vi "CreatePublicEvents.vi"(8 "error in (no error)":errorcluster, 11 "Camera":refnum<class "Camera.lvclass">) -> (0 "error out":errorcluster, 3 "Camera out":refnum<class "Camera.lvclass">)   [LabVIEW 2015, in "Camera.lvclass"]
doc: "---------------------------------------------------------------\nJKI State Machine Objects™\nhttp://jki.net/state-machine-objects/\nCopyright (C) 2005-2015, JKI <info@jki.net>\nALL RIGHTS RESERVEDJKI State Machine Objects (SMO) 1.0.0.5\nJKI - JKI\nCopyright (c) 2016, JKI"
uses:
  Camera.lvclass
  Camera.lvclass/Camera.ctl
  Typedefs/PublicEvents--Camera.NewImage.ctl
  <vilib>/JKI/JKI SMO/SMO/SMO.lvclass
panel:
  # "For instructions on how to use the JKI State Machine Objects, examples and video tutorials, visit:\nhttp://jki.net/state-machine-objects/\n\nJKI State Machine Objects™\nhttp://jki.net/state-machine-objects/\nCopyright (C) 2005-2015, JKI <info@jki.net>\nALL RIGHTS RESERVED"
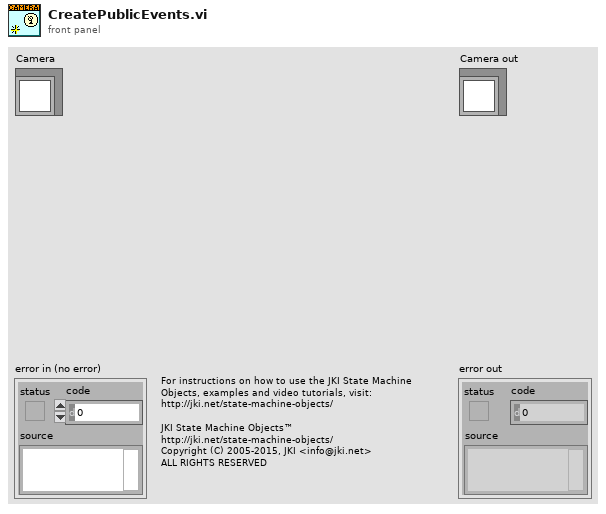
[diagram p1: front panel]
types:
  T1 = typedef "Camera.lvclass/PrivateData--Ref.ctl" = refnum<data-value>
  T2 = typedef "Camera.lvclass/PublicEvents--Camera.NewImage.ctl" = i32
  T3 = typedef "Camera.lvclass/PrivateData--Cluster.ctl" = cluster{"Public Events":T4, "Protected Events":T5, "Private Events":T6, "Dependencies":T7}
  T4 = typedef "Camera.lvclass/PublicEvents--Cluster.ctl" = cluster{"Value Changed":refnum<user-event>, "NewImage":refnum<user-event>, "ImageSaved":refnum<user-event>}
  T5 = typedef "Camera.lvclass/ProtectedEvents--Cluster.ctl" = cluster{"placeholder":refnum<user-event>}
  T6 = typedef "Camera.lvclass/PrivateEvents--Cluster.ctl" = cluster{"New Value":refnum<user-event>, "Grab Image":refnum<user-event>, "Save Image":refnum<user-event>, "Get Image":refnum<user-event>}
  T7 = typedef "Camera.Simulated.lvclass/Dependencies--Cluster.ctl" = cluster{"CircularBuffer.ImageData":refnum<class "CircularBuffer.ImageData.lvclass">}
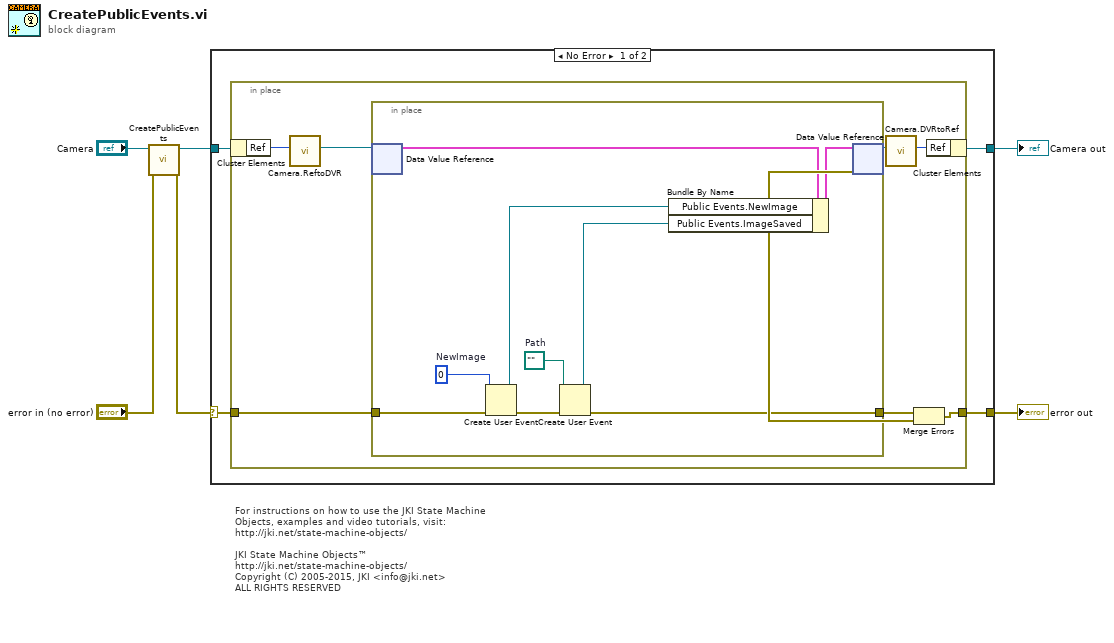
[diagram p0: block diagram]
diagram:
  # "For instructions on how to use the JKI State Machine Objects, examples and video tutorials, visit:\nhttp://jki.net/state-machine-objects/\n\nJKI State Machine Objects™\nhttp://jki.net/state-machine-objects/\nCopyright (C) 2005-2015, JKI <info@jki.net>\nALL RIGHTS RESERVED"
  n1 = call-parent "CreatePublicEvents.vi"("error in (no error)"="error in (no error)", "SMO"="Camera") -> ("error out"=w1:errorcluster, "SMO out"=w3:refnum<class "Camera.lvclass">)  [unwired: 8 in]
  n2 = case shown="No Error" w1 {
    selector: w1 -> [w8 w29]
    tunnel: [w7 w29] -> w5
    tunnel: [w9 w28] -> w6
    tunnel: w3 -> [w10 w28]
    frame No Error {
      n3 = in-place {
        in-place-border: w8 -> [w18]
        in-place-border: [w15] -> w7
        n4 = in-place-cluster #1(w10) -> ("Ref"=w14:u32)
        n5 = call "Camera.ReftoDVR.vi"("Ref"=w14) -> ("Ref"=w13:T1)  [unwired: 10 in]
        n6 = in-place {
          in-place-border: w18 -> [w19]
          in-place-border: [w22] -> w17
          w20 = path ""  # Path
          w24 = T2 0  # NewImage
          n7 = in-place-dvr #2(w13) -> (w26:T3)  [unwired: 1 out]
          n8 = Create User Event(user event datatype=w24, error in=w19) -> (user event=w23:refnum<user-event>, error out=w25:errorcluster)
          n9 = Create User Event(user event datatype=w20, error in=w25) -> (user event=w21:refnum<user-event>, error out=w22:errorcluster)
          n10 = Bundle By Name(cluster=w26, "Public Events.NewImage"=w23, "Public Events.ImageSaved"=w21) -> (w27:T3)
          n11 = in-place-dvr #2(w27) -> (w12:T1, w16:errorcluster)
        }
        n12 = call "Camera.DVRtoRef.vi"("Ref"=w12) -> ("Ref"=w11:u32)  [unwired: 10 in]
        n13 = Merge Errors(w17, w16) -> (w15:errorcluster)
        n14 = in-place-cluster #1("Ref"=w11) -> (w9:refnum<class "Camera.lvclass">)
      }
    }
    frame Error {
    }
  }
  "error out" <- w5
  "Camera out" <- w6
